vi "ProcessVerbosityQueueName.vi"() -> (0 "processVerbosityQueueName":string)   [LabVIEW 2026, in "Lumberjack.lvlib"]
doc: "Returns the fixed process-global named-queue key for the CatchError verbosity store. Shared by SetVerbosity and GetVerbosity so both address the same single-element queue."
uses:
  Lumberjack.lvlib
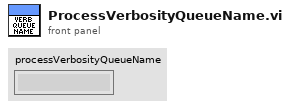
[diagram p1: front panel]
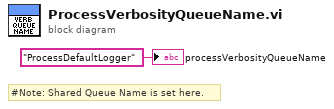
[diagram p0: block diagram]
diagram:
  # "#Note: Shared Queue Name is set here."
  "processVerbosityQueueName" <- "ProcessDefaultLogger" ("processDefaultQueueName")
